vi "Rohde & Schwarz VNA Measure.vi"(5 "Miscellaneous Parameters":T1, 7 "Rohde & Schwarz VNA":T5, 8 "error in (no error)":errorcluster, 9 "SP Stimulus":T2={"Use Instrument Settings"=FALSE, "Blank Frequencies"=FALSE, "Sweep Type"=enum."Linear", "Sweep"={"Fstart"=500.0, "Fstop"=1500.0, "Units"=enum."MHz", "Points"=201}, "Power (dBm)"=999.0, "IFBW (Hz)"=-1.0, "Sweep Time (s)"=-1.0, "Calibration"={"State"=FALSE, "String"=""}} {"Sweep Time (s)" format="%.3g"}, 10 "Parameters to Measure":T6[](array[typedef]) {"Channel" min=1 max=99 step=1; "Parameter"."Stimulus Port" min=1 step=1; "Parameter"."Response Port" min=1 step=1}, 11 "VISA Resource Name":refnum<visa-resource-name>) -> (0 "error out":errorcluster, 1 "S Parameters":cluster{"f0":dbl, "df":dbl, cdb[][]}, 2 "Parameters Measured":T6[](array[typedef]) {"Channel" min=1 max=99 step=1; "Parameter"."Stimulus Port" min=1 step=1; "Parameter"."Response Port" min=1 step=1}, 3 "dup VISA Resource Name":refnum<visa-resource-name>)   [LabVIEW 2011]
uses:
  tests/S Parameter/TypeDefs/SP Parameter to Measure.ctl
  tests/S Parameter/TypeDefs/SP Parameter.ctl
  tests/S Parameter/TypeDefs/SP Calibration State.ctl
  tests/S Parameter/TypeDefs/SP Measurement Format.ctl
  TypeDefs/Rohde & Schwarz VNA Instrument Info.ctl
  tests/S Parameter/TypeDefs/SP Stimulus Parameters.ctl
  tests/S Parameter/TypeDefs/SP Frequency Units.ctl
  tests/S Parameter/TypeDefs/SP Miscellaneous Parameters.ctl
  TypeDefs/Rohde & Schwarz VNA External Trigger Mode.ctl
  TypeDefs/Rohde & Schwarz VNA Measurement.ctl
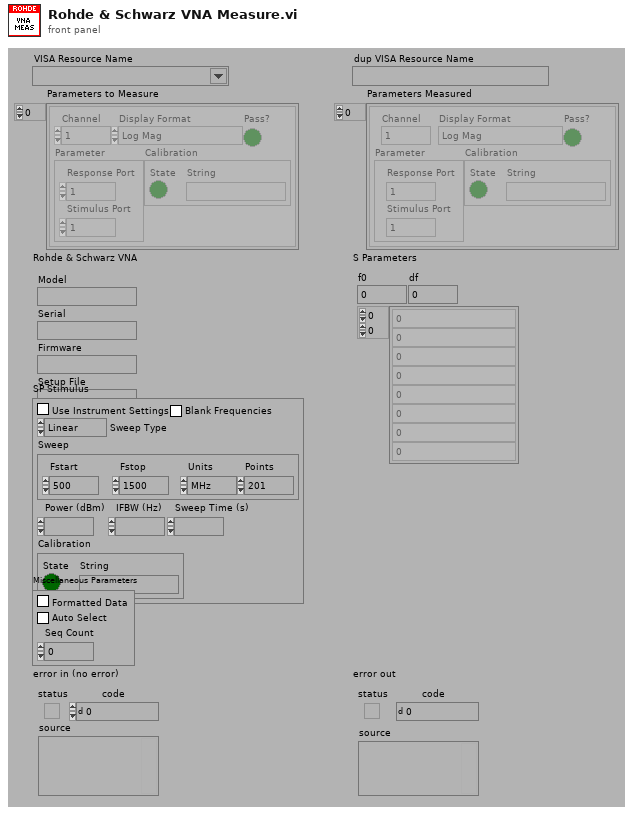
[diagram p1: front panel]
types:
  T1 = typedef "SP Miscellaneous Parameters.ctl" = cluster{"Formatted Data":bool, "Auto Select":bool, "Seq Count":u32}
  T2 = typedef "SP Stimulus Parameters.ctl" = cluster{"Use Instrument Settings":bool, "Blank Frequencies":bool, "Sweep Type":enum32{"Linear", "Logarithmic", "List", "Power", "CW"}, "Sweep":cluster{"Fstart":dbl, "Fstop":dbl, "Units":T3, "Points":i32}, "Power (dBm)":dbl, "IFBW (Hz)":dbl, "Sweep Time (s)":dbl, "Calibration":T4}
  T3 = typedef "SP Frequency Units.ctl" = enum16{"Hz", "kHz", "MHz", "GHz", "Points"}
  T4 = typedef "SP Calibration State.ctl" = cluster{"State":bool, "String":string}
  T5 = typedef "Rohde & Schwarz VNA Instrument Info.ctl" = cluster{"Model":string, "Serial":string, "Firmware":string, "Setup File":string}
  T6 = typedef "SP Parameter to Measure.ctl" = cluster{"Channel":i8, "Parameter":T7, "Calibration":T4, "Display Format":T8, "Pass?":bool}
  T7 = typedef "SP Parameter.ctl" = cluster{"Stimulus Port":i8, "Response Port":i8}
  T8 = typedef "SP Measurement Format.ctl" = enum32{"Log Mag", "Phase", "Delay", "Smith (R+jX)", "Polar (Re/Im)", "Linear Mag", "SWR", "Real", "Imaginary", "Smith (Lin/Phase)", "Smith (Log/Phase)", "Smith (Real/Imag)", "Smith (G+jB)", "Polar (Lin/Phase)", "Polar (Log/Phase)", "Expanded Phase", "Positive Phase", "Inverted Smith", "Unwrapped Phase", "Power Out", "Power In", "Linear Mag/Phase", "Log Mag/Phase", "Real/Imaginary"}
  T9 = typedef "Rohde & Schwarz VNA External Trigger Mode.ctl" = enum16{"Off", "Rising Edge", "Falling Edge", "Periodic", "Manual"}
  T10 = typedef "Rohde & Schwarz VNA Measurement.ctl" = enum32{"S11", "S12", "S21", "S22", "A1 Port 1 Source", "A1 Port 2 Source", "A2 Port 1 Source", "A2 Port 2 Source", "B1 Port 1 Source", "B1 Port 2 Source", "B2 Port 1 Source", "B2 Port 2 Source", "A1/A2 Port 1 Source", "A1/A2 Port 2 Source", "A1/B1 Port 1 Source", "A1/B1 Port 2 Source", "A1/B2 Port 1 Source", "A1/B2 Port 2 Source", "A2/A1 Port 1 Source", "A2/A1 Port 2 Source", "A2/B1 Port 1 Source", "A2/B1 Port 2 Source", "A2/B2 Port 1 Source", "A2/B2 Port 2 Source", "B1/A1 Port 1 Source", "B1/A1 Port 2 Source", "B1/A2 Port 1 Source", "B1/A2 Port 2 Source", "B1/B2 Port 1 Source", "B1/B2 Port 2 Source", "B2/A1 Port 1 Source", "B2/A1 Port 2 Source", "B2/A2 Port 1 Source", "B2/A2 Port 2 Source", "B2/B1 Port 1 Source", "B2/B1 Port 2 Source", "Z<-S11", "Z<-S12", "Z<-S21", "Z<-S22", "Y<-S11", "Y<-S12", "Y<-S21", "Y<-S22", "Z11", "Z12", "Z21", "Z22", "Y11", "Y12", "Y21", "Y22", "DC±1V", "DC±10V", "Unsupported"}
  T11 = typedef "Agilent VNA Measurements.ctl" = cluster{"Channel":i8, "Traces":cluster{"Trace":i8, "Parameter":T7}[]}
  T12 = typedef "Rohde & Schwarz VNA Trigger Mode.ctl" = enum16{"Continuous", "Hold", "Single"}
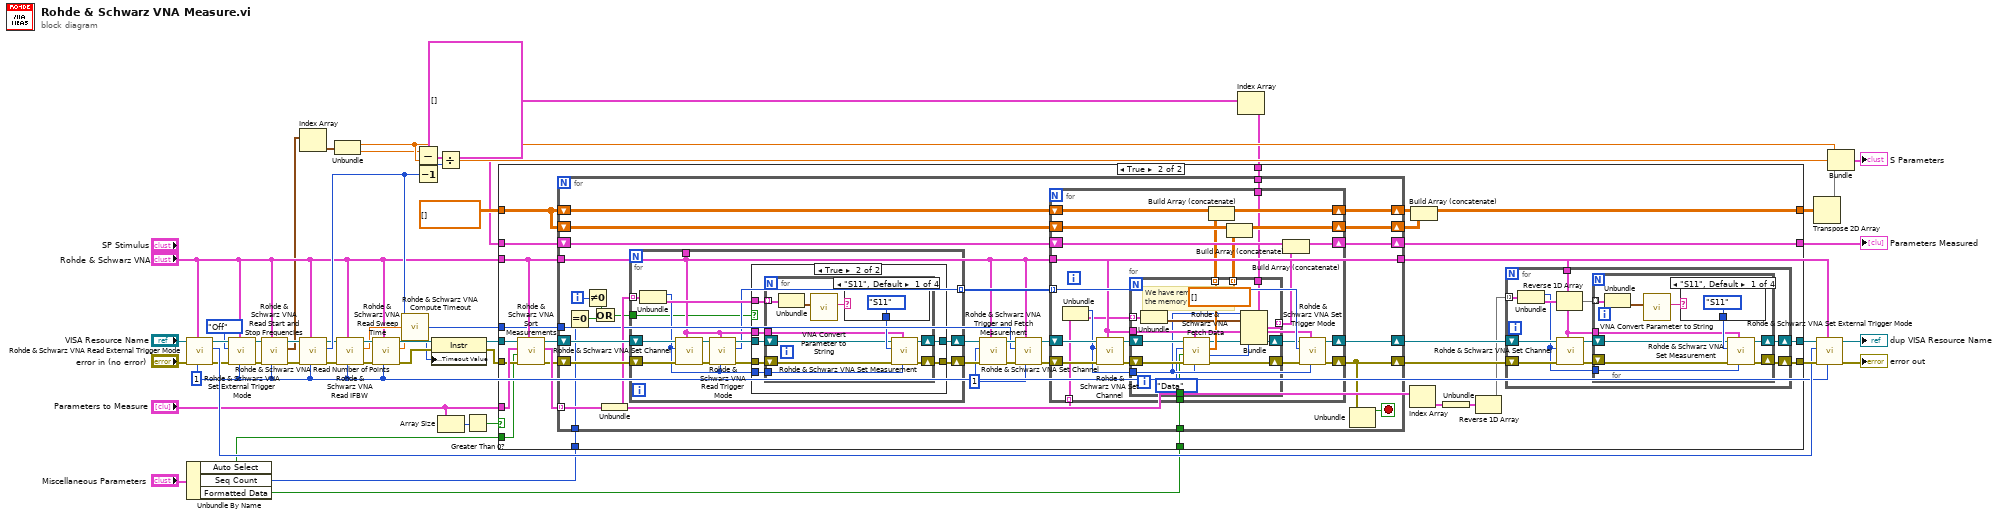
[diagram p0: block diagram]
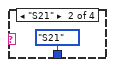
[diagram p4: hidden frame]
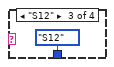
[diagram p5: hidden frame]
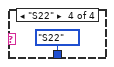
[diagram p6: hidden frame]
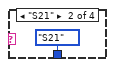
[diagram p7: hidden frame]
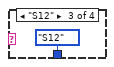
[diagram p8: hidden frame]
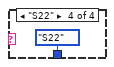
[diagram p9: hidden frame]
diagram:
  w7 = T6[] [] ("Parameters to Measure")
  w11 = i8 1
  n1 = call "Rohde & Schwarz VNA Read External Trigger Mode.vi"("Channel"=w11, "Rohde & Schwarz VNA"="Rohde & Schwarz VNA", "error in (no error)"="error in (no error)", "VISA Resource Name"="VISA Resource Name") -> ("error out"=w33:errorcluster, "Ext. Trigger Mode"=w34:T9, "dup VISA Resource Name"=w32:refnum<visa-resource-name>)  [unwired: 5 out]
  n2 = Unbundle By Name("Miscellaneous Parameters") -> ("Auto Select"=w8:bool, "Seq Count"=w1:u32, "Formatted Data"=w9:bool)
  n3 = call "Rohde & Schwarz VNA Set External Trigger Mode.vi"("Channel"=w11, "Rohde & Schwarz VNA"="Rohde & Schwarz VNA", "error in (no error)"=w33, "Ext. Trigger Mode"=Rohde_&_Schwarz_VNA_External_Trigger_Mode."Off", "VISA Resource Name"=w32) -> ("error out"=w18:errorcluster, "dup VISA Resource Name"=w17:refnum<visa-resource-name>)  [unwired: 5 out]
  n4 = call "Rohde & Schwarz VNA Read Start and Stop Frequencies.vi"("Channel"=w11, "Rohde & Schwarz VNA"="Rohde & Schwarz VNA", "error in (no error)"=w18, "VISA Resource Name"=w17) -> ("error out"=w5:errorcluster, "Start/Stop Freqs, MHz"=w3:cluster{"Fstart":dbl, "Fstop":dbl}[], "dup VISA Resource Name"=w4:refnum<visa-resource-name>)  [unwired: 5 out]
  n5 = Index Array(array=w3) -> (element=w2:cluster{"Fstart":dbl, "Fstop":dbl})  [unwired: 1 in]
  n6 = call "Rohde & Schwarz VNA Read Number of Points.vi"("Channel"=w11, "Rohde & Schwarz VNA"="Rohde & Schwarz VNA", "error in (no error)"=w5, "VISA Resource Name"=w4) -> ("error out"=w15:errorcluster, "Number Points"=w19:i32, "dup VISA Resource Name"=w16:refnum<visa-resource-name>)  [unwired: 5 out]
  n7 = Unbundle(w2) -> ("Fstart"=w40:dbl, "Fstop"=w39:dbl)
  n8 = call "Rohde & Schwarz VNA Read IFBW.vi"("Channel"=w11, "Rohde & Schwarz VNA"="Rohde & Schwarz VNA", "error in (no error)"=w15, "VISA Resource Name"=w16) -> ("error out"=w29:errorcluster, "IFBW, Hz"=w26:dbl, "dup VISA Resource Name"=w30:refnum<visa-resource-name>)  [unwired: 5 out]
  n9 = call "Rohde & Schwarz VNA Read Sweep Time.vi"("Channel"=w11, "Rohde & Schwarz VNA"="Rohde & Schwarz VNA", "error in (no error)"=w29, "VISA Resource Name"=w30) -> ("error out"=w28:errorcluster, "Sweep Time, s"=w25:dbl, "dup VISA Resource Name"=w27:refnum<visa-resource-name>)  [unwired: 5 out]
  n10 = call "Rohde & Schwarz VNA Compute Timeout.vi"("Points"=w19, "IFBW (Hz)"=w26, "Sweep Time (s)"=w25) -> ("Timeout (ms)"=w22:u32)  [unwired: 12 out]
  n11 = Subtract(x=w39, y=w40) -> (x-y=w48:dbl)
  n12 = Decrement(x=w19) -> (x-1=w47:i32)
  n13 = property class="Instr"(reference=w27, error in=w28, "General Settings:Timeout Value"=w22) -> (reference out=w41:refnum<visa-resource-name>, error out=w38:errorcluster)
  n14 = Divide(x=w48, y=w47) -> (x/y=w45:dbl)
  n15 = Array Size(array="Parameters to Measure") -> (size(s)=w43:i32)
  n16 = Greater Than 0?(x=w43) -> (x > 0?=w42:bool)
  n17 = Index Array(array=w7) -> (element=w6:T6)  [unwired: 1 in]
  n18 = case shown="True" w42 {
    tunnel: [w53 w72] -> w36
    tunnel: w41 -> [w51 w59]
    tunnel: "Parameters to Measure" -> [_ w79]
    tunnel: [w52 w64] -> w49
    tunnel: "Rohde & Schwarz VNA" -> [_ w78]
    tunnel: w38 -> [w53 w60]
    tunnel: cdb[][] [] -> [w52 w67]
    tunnel: [w51 w71] -> w35
    tunnel: w22 -> [_ w68]
    tunnel: w9 -> [_ w63]
    tunnel: [w50 w62] -> w12
    tunnel: w7 -> [w50 w61]
    tunnel: w8 -> [_ w56]
    tunnel: w6 -> [_ w55]
    tunnel: w1 -> [_ w54]
    frame False {
    }
    frame True {
      n19 = call "Rohde & Schwarz VNA Sort Measurements.vi"("Rohde & Schwarz VNA"=w78, "error in (no error)"=w60, "Auto Select"=w56, "Parameters to Measure"=w79, "VISA Resource Name"=w59) -> ("error out"=w57:errorcluster, "Sorted Measurements"=w77:cluster{"Measurements":T11[]}[], "dup VISA Resource Name"=w58:refnum<visa-resource-name>)  [unwired: 4 out]
      n20 = for {
        shift-right: [w98] -> w73
        shift-left: w57 -> [w107]
        tunnel: w77 -> [w108] mode=indexing
        tunnel: w78 -> [w87]
        shift-right: [w90] -> w65
        shift-left: w67 -> [w93]
        shift-right: [w99] -> w74
        shift-left: w58 -> [w109]
        tunnel: [w87] -> w69
        tunnel: w68 -> [w96]
        shift-right: [w89] -> w66
        shift-left: w67 -> [w92]
        tunnel: w63 -> [w95]
        shift-right: [w88] -> w62
        shift-left: w61 -> [w91]
        tunnel: w55 -> [w86]
        tunnel: w54 -> [w82]
        i -> [w83]
        stop <- w94 stop-if-true
        w80 = i8 1 ("Channel")
        n21 = Equal To 0?(x=w82) -> (x = 0?=w85:bool)
        n22 = Not Equal To 0?(x=w83) -> (x != 0?=w84:bool)
        n23 = Or(x=w84, y=w85) -> (x .or. y?=w81:bool)
        n24 = Unbundle(w108) -> ("Measurements"=w100:T11[])
        n25 = for {
          tunnel: w87 -> [w152]
          tunnel: w100 -> [w160] mode=indexing
          shift-right: [w158] -> w104
          shift-left: w107 -> [w161]
          shift-right: [w159] -> w103
          shift-left: w109 -> [w162]
          tunnel: [w150] -> w97 mode=indexing
          tunnel: w81 -> [w149]
          n26 = Unbundle(w160) -> ("Channel"=w151:i8, "Traces"=w157:cluster{"Trace":i8, "Parameter":T7}[])
          n27 = call "Rohde & Schwarz VNA Set Channel.vi"("Rohde & Schwarz VNA"=w152, "error in (no error)"=w161, "Channel"=w151, "VISA Resource Name"=w162) -> ("error out"=w155:errorcluster, "dup VISA Resource Name"=w156:refnum<visa-resource-name>)  [unwired: 6 out]
          n28 = call "Rohde & Schwarz VNA Read Trigger Mode.vi"("Channel"=w151, "Rohde & Schwarz VNA"=w152, "error in (no error)"=w155, "VISA Resource Name"=w156) -> ("error out"=w153:errorcluster, "Trigger Mode"=w150:T12, "dup VISA Resource Name"=w154:refnum<visa-resource-name>)  [unwired: 5 out]
          n29 = case shown="True" w149 {
            tunnel: [w164 w171] -> w159
            tunnel: [w163 w170] -> w158
            tunnel: w157 -> [_ w169]
            tunnel: w154 -> [w164 w168]
            tunnel: w153 -> [w163 w167]
            tunnel: w152 -> [_ w166]
            tunnel: w151 -> [_ w165]
            frame False {
              # "Save time because we know that\nthe previous run set these\nmeasurements back to the first\nparameters.  The cannot be skipped\nif it is the second measurement in a\nrun though or if it is the first time\nthrough."
            }
            frame True {
              n30 = for {
                tunnel: w166 -> [w180]
                tunnel: w165 -> [w176]
                tunnel: w169 -> [w175] mode=indexing
                shift-right: [w179] -> w171
                shift-left: w168 -> [w172]
                shift-right: [w178] -> w170
                shift-left: w167 -> [w173]
                n31 = Unbundle(w175) -> ("Parameter"=w174:T7)  [unwired: 1 out]
                n32 = call "VNA Convert Parameter to String.vi"("Parameter"=w174) -> ("Parameter String"=w177:string)  [unwired: 10 out]
                n33 = case shown="\"S11\", Default" w177 {
                  tunnel: [Rohde_&_Schwarz_VNA_Measurement."S11" ("Measurement (S11)") Rohde_&_Schwarz_VNA_Measurement."S21" ("Measurement (S11)") Rohde_&_Schwarz_VNA_Measurement."S12" ("Measurement (S11)") Rohde_&_Schwarz_VNA_Measurement."S22" ("Measurement (S11)")] -> w181
                  frame "S11", Default {
                  }
                  frame "S21" {
                  }
                  frame "S12" {
                  }
                  frame "S22" {
                  }
                }
                n34 = call "Rohde & Schwarz VNA Set Measurement.vi"("Channel"=w176, "Rohde & Schwarz VNA"=w180, "error in (no error)"=w173, "Measurement (S11)"=w181, "VISA Resource Name"=w172) -> ("error out"=w178:errorcluster, "dup VISA Resource Name"=w179:refnum<visa-resource-name>)  [unwired: 1 in, 4 out]
              }
            }
          }
        }
        n35 = call "Rohde & Schwarz VNA Set Channel.vi"("Rohde & Schwarz VNA"=w87, "error in (no error)"=w104, "Channel"=w80, "VISA Resource Name"=w103) -> ("error out"=w102:errorcluster, "dup VISA Resource Name"=w101:refnum<visa-resource-name>)  [unwired: 6 out]
        n36 = call "Rohde & Schwarz VNA Trigger and Fetch Measurement.vi"("Channel"=w80, "Rohde & Schwarz VNA"=w87, "error in (no error)"=w102, "Timout, ms (10000)"=w96, "VISA Resource Name"=w101) -> ("error out"=w106:errorcluster, "dup VISA Resource Name"=w105:refnum<visa-resource-name>)  [unwired: 5 out]
        n37 = for {
          shift-right: [w128] -> w98
          shift-left: w106 -> [w133]
          tunnel: w100 -> [w123] mode=indexing
          shift-right: [w129] -> w99
          shift-left: w105 -> [w132]
          tunnel: w97 -> [w127] mode=indexing
          tunnel: w95 -> [w124]
          shift-right: [w116] -> w88
          shift-left: w91 -> [w119]
          shift-right: [w117] -> w89
          shift-left: w92 -> [w120]
          shift-right: [w118] -> w90
          shift-left: w93 -> [w121]
          tunnel: w87 -> [w113]
          tunnel: w86 -> [w111]
          n38 = Unbundle(w123) -> ("Channel"=w122:i8, "Traces"=w112:cluster{"Trace":i8, "Parameter":T7}[])
          n39 = call "Rohde & Schwarz VNA Set Channel.vi"("Rohde & Schwarz VNA"=w113, "error in (no error)"=w133, "Channel"=w122, "VISA Resource Name"=w132) -> ("error out"=w130:errorcluster, "dup VISA Resource Name"=w131:refnum<visa-resource-name>)  [unwired: 6 out]
          n40 = for {
            tunnel: w124 -> [w145]
            tunnel: w122 -> [w138]
            tunnel: [w144] -> w115 mode=indexing
            tunnel: [cdb[] [] ("Data (real+imag)")] -> w114 mode=indexing
            tunnel: w113 -> [w143]
            shift-right: [w136] -> w125
            shift-left: w130 -> [w147]
            shift-right: [w135] -> w126
            shift-left: w131 -> [w148]
            tunnel: w112 -> [w142] mode=indexing
            tunnel: w111 -> [w140]
            tunnel: [w137] -> w110 mode=indexing
            # "We have removed\nthe memory function."
            n41 = Unbundle(w142) -> ("Parameter"=w139:T7)  [unwired: 1 out]
            n42 = call "Rohde & Schwarz VNA Fetch Data.vi"("Channel"=w138, "Rohde & Schwarz VNA"=w143, "error in (no error)"=w147, "Formatted Data?"=w145, "Data to Read (Data)"=enum16{"Data", "Memory"}."Data", "VISA Resource Name"=w148) -> ("error out"=w136:errorcluster, "Display Format"=w141:T8, "Data (real+imag)"=w144:cdb[], "dup VISA Resource Name"=w135:refnum<visa-resource-name>)  [unwired: 2 out]
            n43 = Bundle(cluster=w140, "Channel"=w138, "Parameter"=w139, "Display Format"=w141) -> (w137:T6)  [unwired: 2 out]
          }
          n44 = Build Array (concatenate)(w121, w115) -> (w118:cdb[][])
          n45 = Build Array (concatenate)(w120, w114) -> (w117:cdb[][])
          n46 = Build Array (concatenate)(w119, w110) -> (w116:T6[])
          n47 = call "Rohde & Schwarz VNA Set Trigger Mode.vi"("Channel"=w122, "Rohde & Schwarz VNA"=w113, "error in (no error)"=w125, "Trigger Mode"=w127, "VISA Resource Name"=w126) -> ("error out"=w128:errorcluster, "dup VISA Resource Name"=w129:refnum<visa-resource-name>)  [unwired: 5 out]
        }
        n48 = Unbundle(w98) -> ("status"=w94:bool)  [unwired: 2 out]
      }
      n49 = Index Array(array=w77) -> (element=w76:cluster{"Measurements":T11[]})  [unwired: 1 in]
      n50 = Build Array (concatenate)(w65, w66) -> (w64:cdb[][])
      n51 = Unbundle(w76) -> ("Measurements"=w75:T11[])
      n52 = Reverse 1D Array(array=w75) -> (reversed array=w70:T11[])
      n53 = for {
        tunnel: w69 -> [w190]
        tunnel: w70 -> [w188] mode=indexing
        shift-right: [w193] -> w72
        shift-left: w73 -> [w195]
        shift-right: [w194] -> w71
        shift-left: w74 -> [w196]
        n54 = Unbundle(w188) -> ("Channel"=w186:i8, "Traces"=w189:cluster{"Trace":i8, "Parameter":T7}[])
        n55 = Reverse 1D Array(array=w189) -> (reversed array=w187:cluster{"Trace":i8, "Parameter":T7}[])
        n56 = call "Rohde & Schwarz VNA Set Channel.vi"("Rohde & Schwarz VNA"=w190, "error in (no error)"=w195, "Channel"=w186, "VISA Resource Name"=w196) -> ("error out"=w192:errorcluster, "dup VISA Resource Name"=w191:refnum<visa-resource-name>)  [unwired: 6 out]
        n57 = for {
          tunnel: w190 -> [w201]
          tunnel: w187 -> [w198] mode=indexing
          shift-right: [w206] -> w194
          shift-left: w191 -> [w202]
          shift-right: [w205] -> w193
          shift-left: w192 -> [w203]
          tunnel: w186 -> [w199]
          n58 = Unbundle(w198) -> ("Parameter"=w197:T7)  [unwired: 1 out]
          n59 = call "VNA Convert Parameter to String.vi"("Parameter"=w197) -> ("Parameter String"=w200:string)  [unwired: 10 out]
          n60 = case shown="\"S11\", Default" w200 {
            tunnel: [Rohde_&_Schwarz_VNA_Measurement."S11" ("Measurement (S11)") Rohde_&_Schwarz_VNA_Measurement."S21" ("Measurement (S11)") Rohde_&_Schwarz_VNA_Measurement."S12" ("Measurement (S11)") Rohde_&_Schwarz_VNA_Measurement."S22" ("Measurement (S11)")] -> w204
            frame "S11", Default {
            }
            frame "S21" {
            }
            frame "S12" {
            }
            frame "S22" {
            }
          }
          n61 = call "Rohde & Schwarz VNA Set Measurement.vi"("Channel"=w199, "Rohde & Schwarz VNA"=w201, "error in (no error)"=w203, "Measurement (S11)"=w204, "VISA Resource Name"=w202) -> ("error out"=w205:errorcluster, "dup VISA Resource Name"=w206:refnum<visa-resource-name>)  [unwired: 1 in, 4 out]
        }
      }
    }
  }
  "Parameters Measured" <- w12
  n62 = Transpose 2D Array(2D array=w49) -> (transposed array=w44:cdb[][])
  n63 = call "Rohde & Schwarz VNA Set External Trigger Mode.vi"("Channel"=w11, "Rohde & Schwarz VNA"="Rohde & Schwarz VNA", "error in (no error)"=w36, "Ext. Trigger Mode"=w34, "VISA Resource Name"=w35) -> ("error out"=→"error out":errorcluster, "dup VISA Resource Name"=→"dup VISA Resource Name":refnum<visa-resource-name>)  [unwired: 5 out]
  n64 = Bundle("Fstart"=w40, w45, w44) -> (→"S Parameters":cluster{"Fstart":dbl, dbl, cdb[][]})  [unwired: 1 out]
